vi "Simulated_Robot_Diff_Drive.vi"() -> ()   [LabVIEW 2019]
doc: "This WebSockets API example VI acts as a server for an incoming websockets connection. Receives/sends string data to the connected client."
uses:
  <vilib>/Rock Robotics/WPI/Simulation/Protocol/Devices/PWM/PWM proto.ctl
  <vilib>/Rock Robotics/WPI/Simulation/Protocol/Devices/PWM/PWM data proto.ctl
  <vilib>/Rock Robotics/WPI/Simulation/Protocol/Devices/RoboRIO/RoboRIO proto.ctl
  <vilib>/Rock Robotics/WPI/Simulation/Protocol/Devices/RoboRIO/RoboRIO data proto.ctl
  <vilib>/Rock Robotics/WPI/Simulation/Protocol/Devices/DriverStation/DS proto.ctl
  <vilib>/Rock Robotics/WPI/Simulation/Protocol/Devices/DriverStation/DS data proto.ctl
  <vilib>/Rock Robotics/WPI/Simulation/Protocol/Devices/Gyro/Gyro proto.ctl
  <vilib>/Rock Robotics/WPI/Simulation/Protocol/Devices/Gyro/Gyro Data proto.ctl
  <vilib>/Rock Robotics/WPI/Simulation/Protocol/Devices/Encoder/Encoder proto.ctl
  <vilib>/Rock Robotics/WPI/Simulation/Protocol/Devices/Encoder/Encoder data protoo.ctl
  <vilib>/Rock Robotics/WPI/ThirdParty/JAS_Junk/TrajLib/TypeDef/DIFF_DRIVE_TRAIN_SIM.ctl
  <vilib>/Rock Robotics/WPI/ThirdParty/JAS_Junk/TrajLib/TypeDef/LINEAR_SYSTEM.ctl
  <vilib>/Analysis/Matrix/Datatypes/RealMatrix.ctl
  <vilib>/Rock Robotics/WPI/ThirdParty/JAS_Junk/TrajLib/TypeDef/DCMOTOR.CTL
  <vilib>/vision/Image Controls.llb/IMAQ Image.ctl
  Simulated_Field/Simulated_Field_ROBOT_PICTURE.ctl
  DiffDriveSim/DiffDriveSim_PhysRobotInfoType.ctl
  DiffDriveSim/DiffDriveSim_KitBotDriveInfoType.ctl
  <vilib>/Rock Robotics/WPI/ThirdParty/JAS_Junk/TrajLib/Enum/DIFF_DRIVE_ToughBoxMini_MotorChoice_ENUM.ctl
  <vilib>/Rock Robotics/WPI/ThirdParty/JAS_Junk/TrajLib/Enum/DIFF_DRIVE_KitBot_WheelSize_ENUM.ctl
  <vilib>/Rock Robotics/WPI/ThirdParty/JAS_Junk/TrajLib/Enum/DIFF_DRIVE_ToughBoxMini_GearChoice_ENUM.ctl
  DiffDriveSim/DiffDriveSim_CustomDriveIntoType.ctl
  <vilib>/Rock Robotics/WPI/ThirdParty/JAS_Junk/TrajLib/Enum/DCMOTOR_TYPES_ENUM.ctl
  DiffDriveSim/DiffDriveSim_EncoderDIOType.ctl
  <vilib>/Rock Robotics/SystemInterfaces/DIO/FPGA_DIOChannel.ctl
  <vilib>/Rock Robotics/SystemInterfaces/DIO/FPGA_DIOPWMChannel.ctl
  <vilib>/Utility/miscctls.llb/LVBoundsTypeDef.ctl
  <vilib>/Rock Robotics/WPI/Simulation/Protocol/Devices/RoboRIO/RoboRIO Update Ops.ctl
  <vilib>/Rock Robotics/WPI/Simulation/Protocol/Devices/DriverStation/DS Update Ops.ctl
  <vilib>/Rock Robotics/WPI/ThirdParty/JAS_Junk/TrajLib/Rotation2d_CreateAngle.vi
  <vilib>/Rock Robotics/WPI/ThirdParty/JAS_Junk/TrajLib/Translation2d_Create.vi
  <vilib>/Rock Robotics/WPI/ThirdParty/JAS_Junk/TrajLib/MathUtil_Clamp.vi
  <vilib>/MediaMongrels Ltd/WebSockets/WebSockets/WebSocket Server/WebSocket Server.lvclass
  C:/Program Files/National Instruments/LabVIEW 2019/vi.lib/MediaMongrels Ltd/WebSockets/WebSockets/WebSocket/WebSocket.lvclass
  <vilib>/picture/pixmap.llb/Flatten Pixmap.vi
  <vilib>/picture/pictutil.llb/Create Mask.vi
  <vilib>/picture/picture.llb/Draw Flattened Pixmap.vi
  Simulated_Field/Simulated_Field.lvlib
  <vilib>/Rock Robotics/WPI/ThirdParty/JAS_Junk/TrajLib/Trajectory_Library.lvlib
  <vilib>/Analysis/Matrix/NI_Matrix.lvlib
panel:
  in  "Tab Control":T1(tab)
  in  "Start Simulation":bool
  in  "Field Selector":string(combo)
  in  "Robot Y Position\nInches":dbl=84.0
  in  "Robot X Position\nInches":dbl=120.0
  in  "Robot Orientation\nDegrees":dbl
  in  "Custom Drive Info":T2={"Motor Type"=enum."CIM", "Num Motors Per Side"=1, "Wheel Diameter Inch"=7.0, "Gear Ratio"=1.0} {"Gear Ratio" format="%#_13g"; "Wheel Diameter Inch" format="%#_13g"}
  in  "Robot Physical Info":T4={"Mass_LB"=80.0, "Actual TrackWidth Inch"=26.0, "Skid Factor"=1.75} {"Actual TrackWidth Inch" format="%#_13g"}
  in  "KitBot Drive Info":T5={"ToughBoxMiniMotor"=enum."One CIM Per Side", "Wheelsize"=enum."6 Inch", "ToughBoxMiniGear"=enum."Ratio_8_45"}
  in  "Use Custom Drive":bool
  in  "Encoder Counts/Rev":dbl=360.0
  in  "Left Drive Encoder":T9={"Enc A DI Channel"=enum."DIO 4", "Enc B DI Channel"=enum."DIO 5"}
  in  "Right Drive Encoder":T9={"Enc A DI Channel"=enum."DIO 6", "Enc B DI Channel"=enum."DIO 7"}
  in  "Left Drive Motor":T11
  in  "Right Drive Motor":T11=enum."PWM 1"
  out "Right Dist Ft":dbl format="%15.1f"
  out "Left Dist Ft":dbl format="%15.1f"
  out "Heading Deg":dbl format="%11.1f"
  out "Right Wheel\nFt / Sec":dbl format="%11.1f"
  out "Left Wheel\nFt / Sec":dbl format="%11.1f"
  out "RSL ON":picture
  out "ROBOT":T12
  out "RSL OFF":picture
  out "Field Picture":picture
  out "Y Pos Inch":dbl format="%11.1f"
  out "X Pos Inch":dbl format="%11.1f"
  out "Gyro":T13={"type"="Gyro", "device"="", "name"="", "data"={"<init"=0, ">connected"=FALSE, "<offsetX"=0.0, "<offsetY"=0.0, "<offsetZ"=0.0, ">angle_x"=0.0, ">angle_y"=0.0, ">angle_z"=0.0, ">rate_x"=0.0, ">rate_y"=0.0, ">rate_z"=0.0, "<gain"=0.0}}
  out "Enc Left":T15={"type"="Encoder", "device"="", "name"="", "data"={"<init"=FALSE, ">count"=0.0, ">period"=0.0, "<samples_to_avg"=0, "<offset"=0.0, "<channel_a"=0, "<channel_b"=0}}
  out "Enc Right":T15={"type"="Encoder", "device"="", "name"="", "data"={"<init"=FALSE, ">count"=0.0, ">period"=0.0, "<samples_to_avg"=0, "<offset"=0.0, "<channel_a"=0, "<channel_b"=0}}
  out "PWM 0":T17
  out "PWM 1":T17
  out "roboRIO":T19={"type"="roboRIO", "device"="", "name"="", "data"={">fpga_button"=FALSE, ">vin_voltage"=0.0, ">vin_current"=0.0, ">6v_voltage"=0.0, ">6v_current"=0.0, ">6v_active"=FALSE, ">6v_faults"=0.0, ">5v_voltage"=0.0, ">5v_current"=0.0, ">5v_active"=FALSE, ">5v_faults"=0.0, ">3v3_voltage"=0.0, ">3v3_current"=0.0, ">3v3_active"=FALSE, ">3v3_faults"=0.0}}
  out "Driverstation":T21={"type"="Driverstation", "device"="", "name"="", "data"={">enabled"=FALSE, ">autonomous"=FALSE, ">test"=FALSE, ">estop"=FALSE, ">fms"=FALSE, ">ds"=FALSE, "<match_time"=0.0, ">station"="", ">game_data"=""}}
  out "Request URI":string
  out "HTTP Headers":variant
  out "Stop Sim":bool
  out "Battery Voltage VDC":dbl format="%18.2f"
  out "Gyro Reading   Deg":dbl format="%19.3f"
  out "Edges/Feet":dbl
  out "out DiffDriveTrainSim":T23 {"m_Motor"."Jr_KgM2" format="%13.5p"; "m_Motor"."L_H" format="%13.5p"; "m_Motor"."Kt_NMPerAmp" format="%13.5p"; "m_Motor"."KvINV_RadPerSecPerVolt" format="%13.5p"; "m_Motor"."R_Ohms" format="%13.5p"; "m_Motor"."FreeSpeed_RadPerSec" format="%13.5p"; "m_Motor"."FreeCurrent_Amps" format="%13.5p"; "m_Motor"."StallCurrent_Amps" format="%13.5p"; "m_Motor"."StallTorque_NM" format="%13.5p"; "m_Motor"."nominalVoltage_Volts" format="%13.5p"}
  out "Speed Left  Ft/Sec":dbl format="%13.2f"
  out "Speed Right  Ft/Sec":dbl format="%13.2f"
  out "Amps":dbl
  out "PWM 0 Rate":dbl format="%19.3f"
  out "PWM 1 Rate":dbl format="%19.3f"
  out "FIeld Image":T27
  out "Y Pos Pixel":dbl format="%11.1f"
  out "X Pos Pixel":dbl format="%11.1f"
  in  "Restart":bool
  out "Ctrl Loop Offset MS":dbl
  out "Robot Enabled":bool
  # "Robot Position"
  # "Robot Speed / Distance"
  # "<States, 1>"
  # "<Outputs, 1>"
  # "<Inputs, 1>"
  # "<Outputs, 1>"
  # "<States,States>"
  # "<States,Inputs>"
  # "<Outputs,States>"
  # "<Outputs,Inputs>"
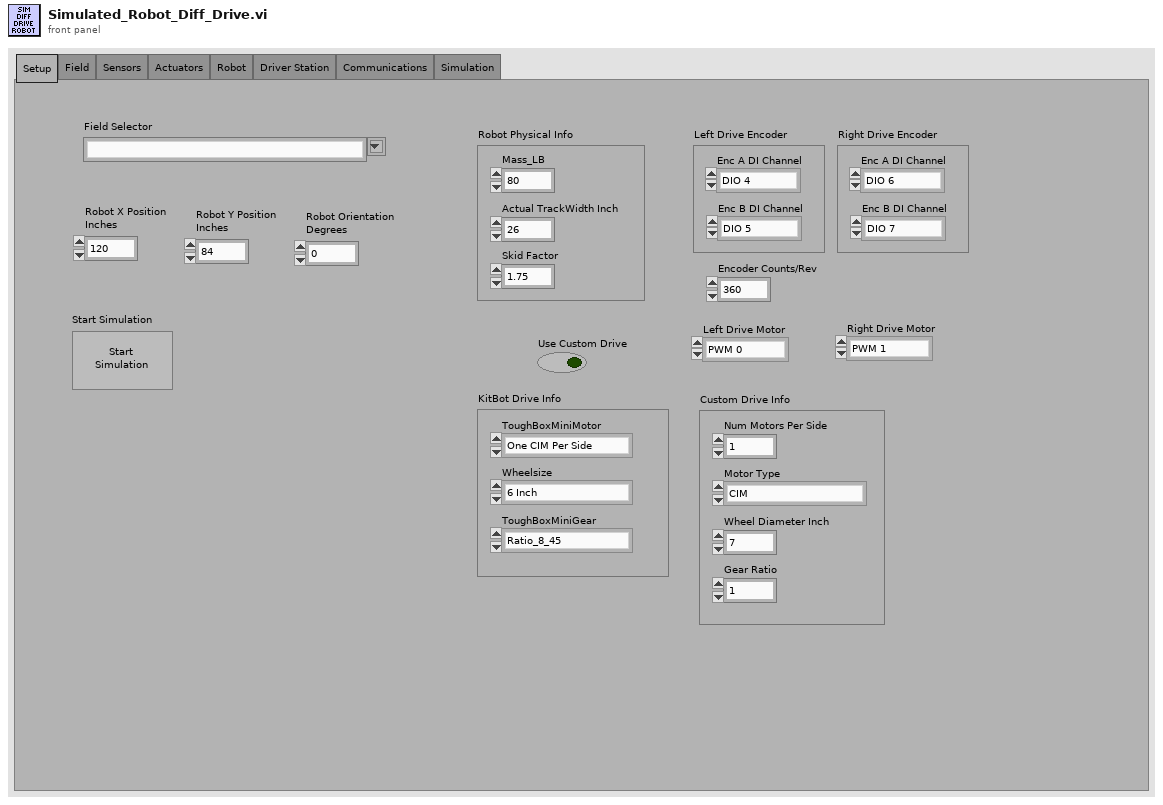
[diagram p1: front panel]
types:
  T1 = enum32{"Setup", "Field", "Sensors", "Actuators", "Robot", "Driver Station", "Communications", "Simulation"}
  T2 = typedef "DiffDriveSim_CustomDriveIntoType.ctl" = cluster{"Motor Type":T3, "Num Motors Per Side":i32, "Wheel Diameter Inch":dbl, "Gear Ratio":dbl}
  T3 = typedef "Trajectory_Library.lvlib/DCMOTOR_TYPES_ENUM.ctl" = enum16{"CIM", "AndyMark 9015", "Andy Mark RS 775 125", "Bag", "BaneBots RS 550", "BaneBots RS 775", "Falcon 500", "Mini CIM", "NEO", "NEO 550", "Romi BuiltIn", "Vex 775 Pro"}
  T4 = typedef "DiffDriveSim_PhysRobotInfoType.ctl" = cluster{"Mass_LB":dbl, "Actual TrackWidth Inch":dbl, "Skid Factor":dbl}
  T5 = typedef "DiffDriveSim_KitBotDriveInfoType.ctl" = cluster{"ToughBoxMiniMotor":T6, "Wheelsize":T7, "ToughBoxMiniGear":T8}
  T6 = typedef "Trajectory_Library.lvlib/DIFF_DRIVE_ToughBoxMini_MotorChoice_ENUM.ctl" = enum16{"One CIM Per Side", "Two CIM Per Side", "One MiniCIM Per Side", "Two Mini CIM Per Side", "Two Falcon Per Side", "Two NEO Per Side"}
  T7 = typedef "Trajectory_Library.lvlib/DIFF_DRIVE_KitBot_WheelSize_ENUM.ctl" = enum16{"4 Inch", "6 Inch", "8 Inch", "10 Inch"}
  T8 = typedef "Trajectory_Library.lvlib/DIFF_DRIVE_ToughBoxMini_GearChoice_ENUM.ctl" = enum16{"Ratio_12_75", "Ratio_10_71", "Ratio_8_45", "Ratio_7_31", "Ratio_5_95"}
  T9 = typedef "DiffDriveSim_EncoderDIOType.ctl" = cluster{"Enc A DI Channel":T10, "Enc B DI Channel":T10}
  T10 = typedef "FPGA_DIOChannel.ctl" = enum8{"DIO 0", "DIO 1", "DIO 2", "DIO 3", "DIO 4", "DIO 5", "DIO 6", "DIO 7", "DIO 8", "DIO 9", "DIO MXP 0", "DIO MXP 1", "DIO MXP 2", "DIO MXP 3", "DIO MXP 4", "DIO MXP 5", "DIO MXP 6", "DIO MXP 7", "DIO MXP 8", "DIO MXP 9", "DIO MXP 10", "DIO MXP 11", "DIO MXP 12", "DIO MXP 13", "DIO MXP 14", "DIO MXP 15", "SPI Port CS1", "SPI Port CS2", "SPI Port CS3", "SPI Port MISO", "SPI Port MOSI", "Invalid"}
  T11 = typedef "FPGA_DIOPWMChannel.ctl" = enum8{"PWM 0", "PWM 1", "PWM 2", "PWM 3", "PWM 4", "PWM 5", "PWM 6", "PWM 7", "PWM 8", "PWM 9", "PWM MXP 0", "PWM MXP 1", "PWM MXP 2", "PWM MXP 3", "PWM MXP 4", "PWM MXP 5", "PWM MXP 6", "PWM MXP 7", "PWM MXP 8", "PWM MXP 9", "Invalid"}
  T12 = typedef "Simulated_Field.lvlib/Simulated_Field_ROBOT_PICTURE.ctl" = picture
  T13 = typedef "Gyro proto.ctl" = cluster{"type":string, "device":string, "name":string, "data":T14}
  T14 = typedef "Gyro Data proto.ctl" = cluster{"<init":i32, ">connected":bool, "<offsetX":dbl, "<offsetY":dbl, "<offsetZ":dbl, ">angle_x":dbl, ">angle_y":dbl, ">angle_z":dbl, ">rate_x":dbl, ">rate_y":dbl, ">rate_z":dbl, "<gain":dbl}
  T15 = typedef "Encoder proto.ctl" = cluster{"type":string, "device":string, "name":string, "data":T16}
  T16 = typedef "Encoder data protoo.ctl" = cluster{"<init":bool, ">count":dbl, ">period":dbl, "<samples_to_avg":i32, "<offset":dbl, "<channel_a":i32, "<channel_b":i32}
  T17 = typedef "PWM proto.ctl" = cluster{"type":string, "device":string, "name":string, "data":T18}
  T18 = typedef "PWM data proto.ctl" = cluster{"<init":bool, "<speed":dbl, "<position":dbl, "<raw":dbl, "<period_scale":dbl, "<zero_latch":bool, "<servo range":dbl}
  T19 = typedef "RoboRIO proto.ctl" = cluster{"type":string, "device":string, "name":string, "data":T20}
  T20 = typedef "RoboRIO data proto.ctl" = cluster{">fpga_button":bool, ">vin_voltage":dbl, ">vin_current":dbl, ">6v_voltage":dbl, ">6v_current":dbl, ">6v_active":bool, ">6v_faults":dbl, ">5v_voltage":dbl, ">5v_current":dbl, ">5v_active":bool, ">5v_faults":dbl, ">3v3_voltage":dbl, ">3v3_current":dbl, ">3v3_active":bool, ">3v3_faults":dbl}
  T21 = typedef "DS proto.ctl" = cluster{"type":string, "device":string, "name":string, "data":T22}
  T22 = typedef "DS data proto.ctl" = cluster{">enabled":bool, ">autonomous":bool, ">test":bool, ">estop":bool, ">fms":bool, ">ds":bool, "<match_time":dbl, ">station":string, ">game_data":string}
  T23 = typedef "Trajectory_Library.lvlib/DIFF_DRIVE_TRAIN_SIM.ctl" = cluster{"m_Plant":T24, "m_X":T25, "m_Y":T25, "m_U":T25, "MeasureStdDev":T25, "m_Motor":T26, "m_OriginalGearing":dbl, "m_CurrentGearing":dbl, "m_WheelRadius_M":dbl, "m_RB":dbl}
  T24 = typedef "Trajectory_Library.lvlib/LINEAR_SYSTEM.ctl" = cluster{"m_A":T25, "m_B":T25, "m_C":T25, "m_D":T25, "States":i32, "Inputs":i32, "Outputs":i32}
  T25 = typedef "NI_Matrix.lvlib/RealMatrix.ctl" = dbl[][]
  T26 = typedef "Trajectory_Library.lvlib/DCMOTOR.CTL" = cluster{"nominalVoltage_Volts":dbl, "StallTorque_NM":dbl, "StallCurrent_Amps":dbl, "FreeCurrent_Amps":dbl, "FreeSpeed_RadPerSec":dbl, "R_Ohms":dbl, "KvINV_RadPerSecPerVolt":dbl, "Kt_NMPerAmp":dbl, "L_H":dbl, "Jr_KgM2":dbl}
  T27 = typedef "IMAQ Image.ctl" = refnum<image>
  T28 = typedef "LVBoundsTypeDef.ctl" = cluster{"Width":u32, "Height":u32}
  T29 = typedef "Image Type" = u32
  T30 = typedef "Simulated_Field.lvlib/Simulated_Field_Field_Info.ctl" = cluster{"FIeld_File_Name":string, "Top_Left_X":i32, "Top_Left_Y":i32, "Bottom_Right_X":i32, "Bottom_Right_Y":i32, "Field_Size_X":dbl, "Field_Size_Y":dbl, "FIeld_Size_Units":string}
  T31 = typedef "Trajectory_Library.lvlib/POSE2D.ctl" = cluster{"TRANSLATION":T32, "ROTATION":T33}
  T32 = typedef "Trajectory_Library.lvlib/TRANSLATION2D.ctl" = cluster{"X":dbl, "Y":dbl}
  T33 = typedef "Trajectory_Library.lvlib/ROTATION2D.ctl" = cluster{"VALUE":dbl, "COS":dbl, "SIN":dbl}
  T34 = typedef "Simulated_Field.lvlib/Simulated_FIeld_Rotated_Picture_TypeDef.ctl" = cluster{"ONE-8-bit pixmap":u8[][], "Two-Array":cdb[][], "Three-Numeric":i32, "Four-Numeric":i32, "Five-Numeric":cdb, "Six-colors":u32[], "Seven-new element/subarray":u32, "Eight-Cluster":cluster{"[0]":i32, "[1]":i32}}
  T35 = typedef "DS Update Ops.ctl" = enum16{"set enabled", "set autonomous", "set test", "set estop", "set fms", "set ds", "set control word", "set match_time", "set station", "set game data", "JSON update", "set name", "get", "transmit initial", "reset"}
  T36 = typedef "RoboRIO Update Ops.ctl" = enum16{"get", "JSON update", "set name", "transmit initial", "set fpga_button", "set vin_voltage", "set vin_current", "set 6v_voltage", "set 6v_current", "set 6v_active", "set 6v_faults", "set 5v_voltage", "set 5v_current", "set 5v_active", "set 5v_faults", "set 3v3_voltage", "set 3v3_current", "set 3v3_active", "set 3v3_faults", "reset"}
  T37 = cluster{"Right Speed Ft/Sec":dbl, "Right Distance Ft":dbl}
  T38 = cluster{"Left Speed Ft/Sec":dbl, "Left Distance Ft":dbl}
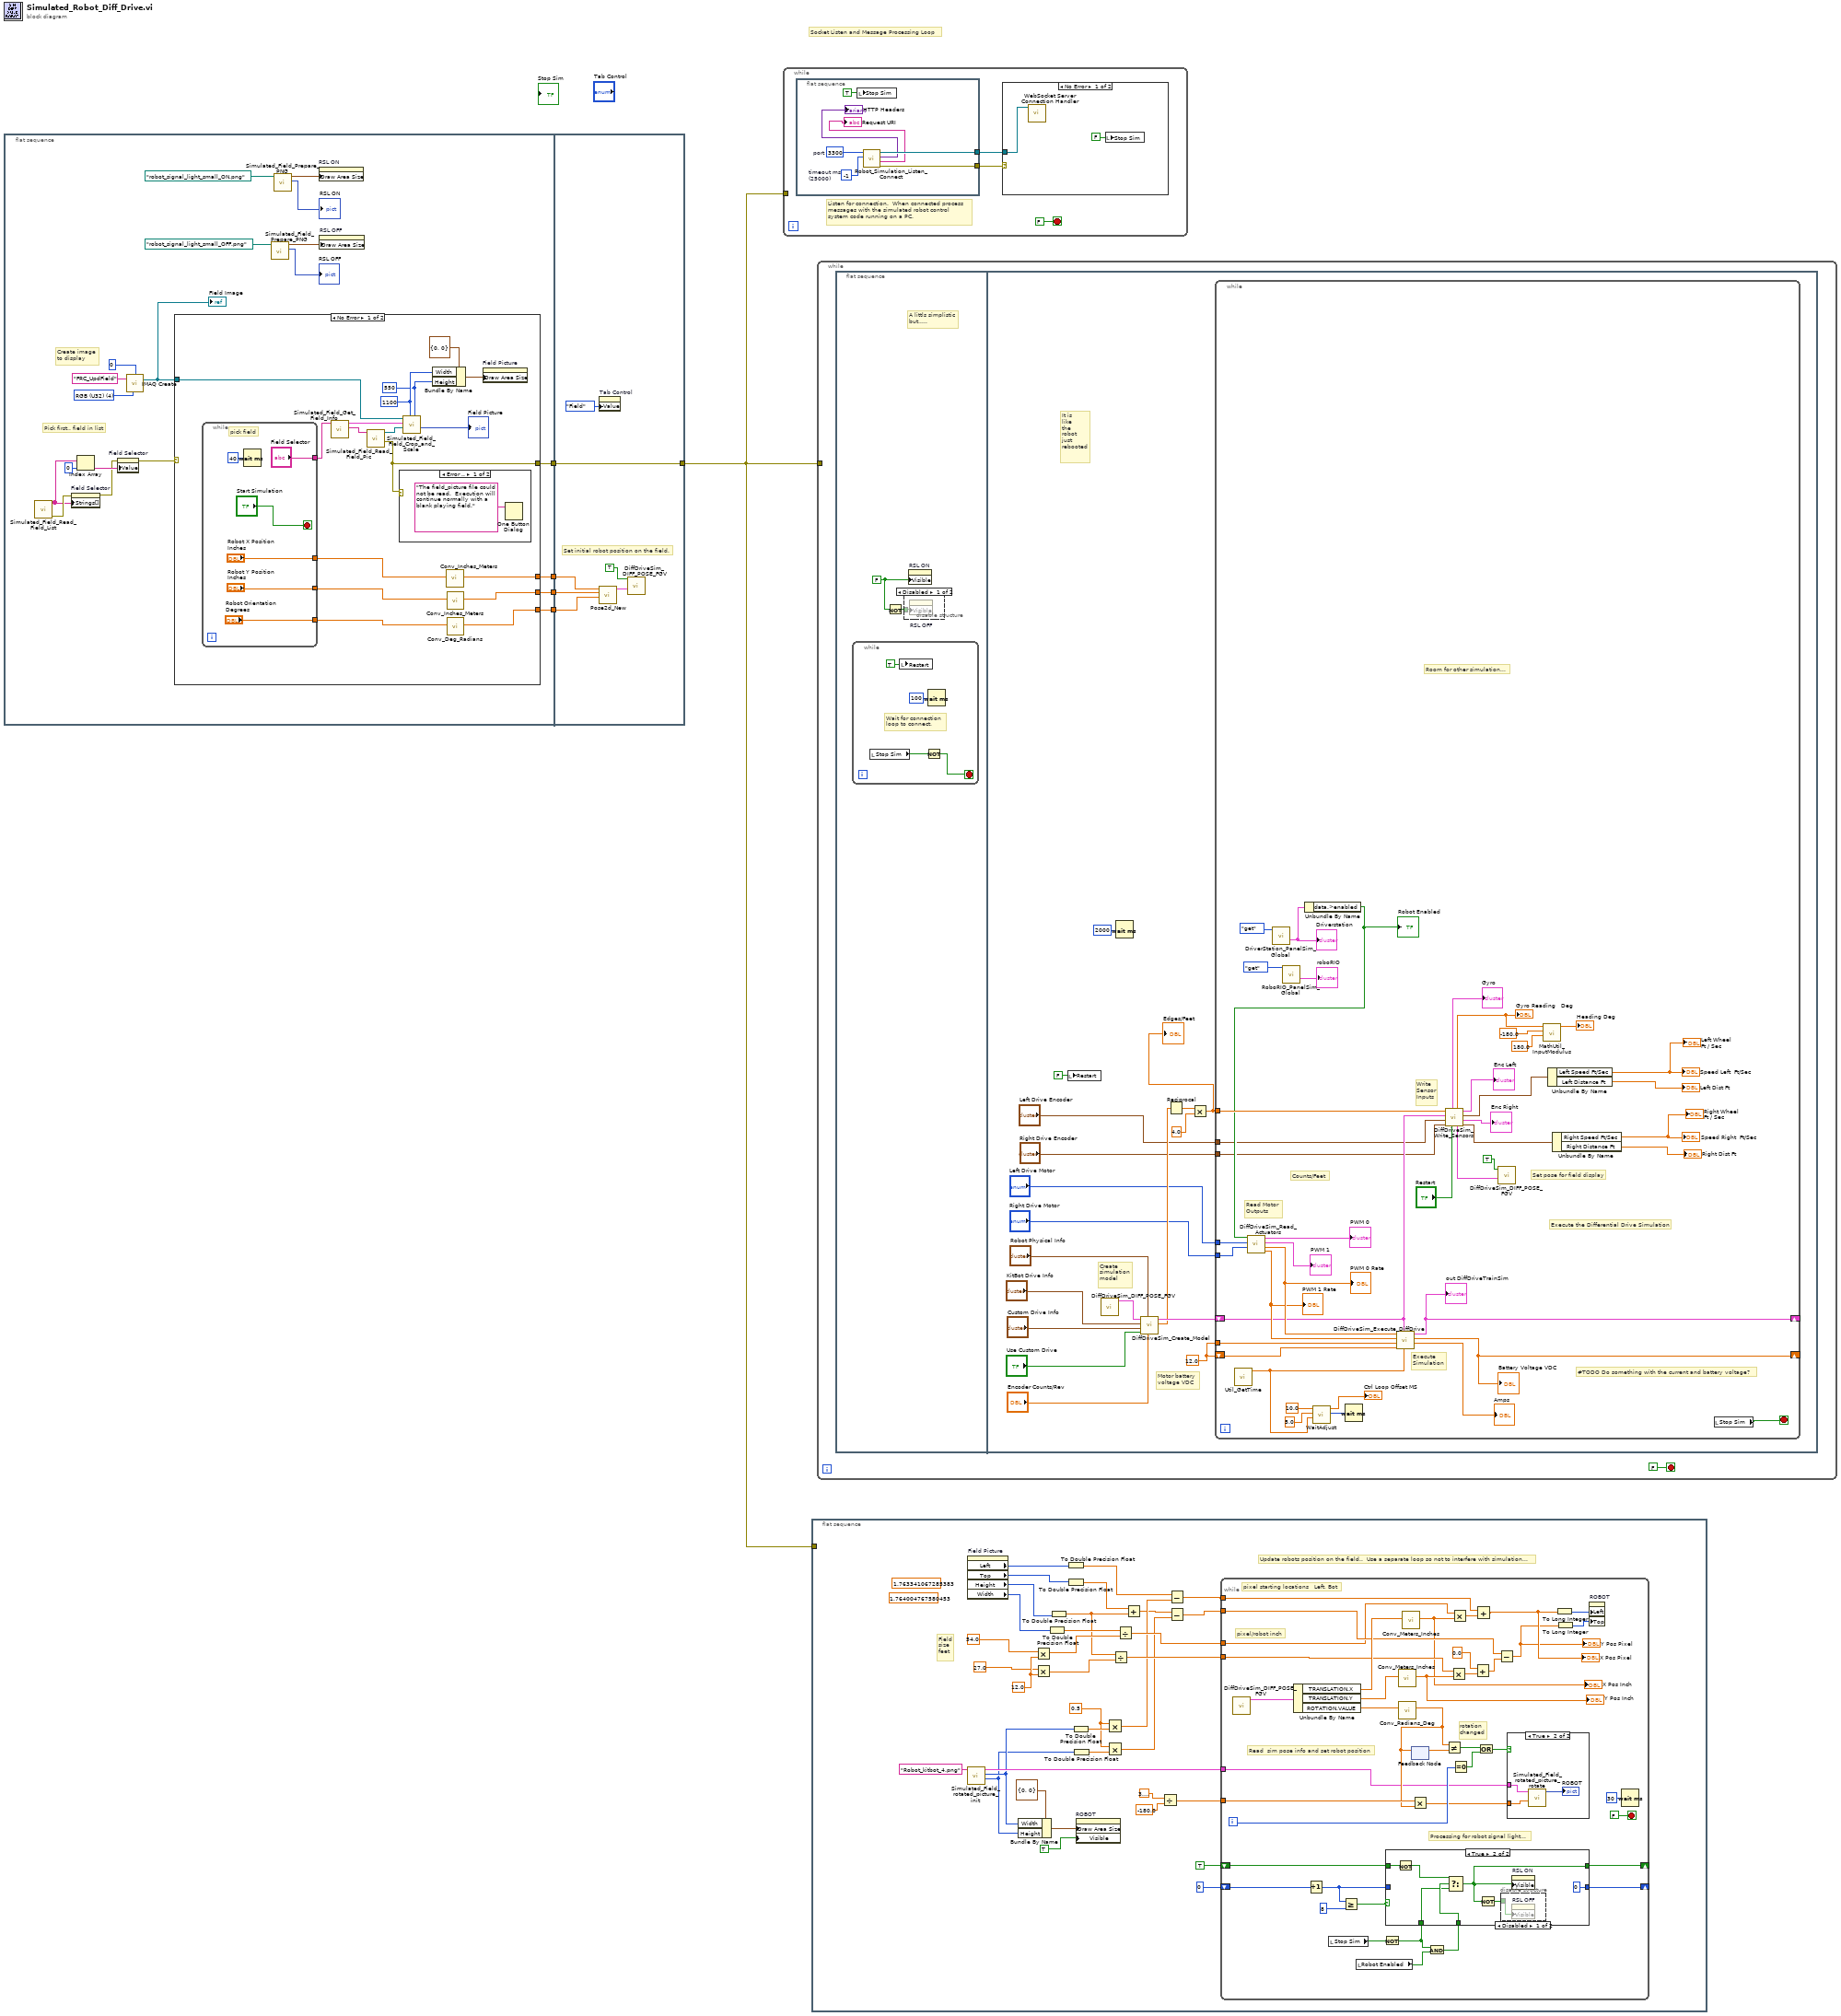
[diagram p0: block diagram]
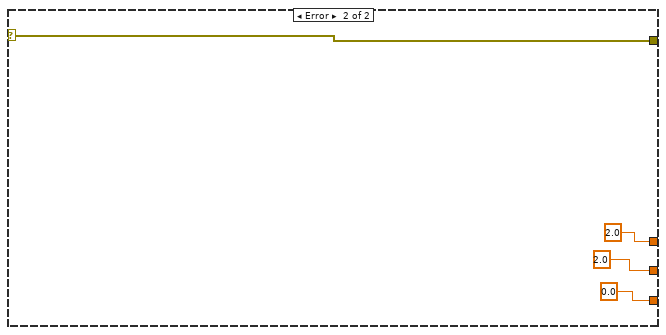
[diagram p6: hidden frame]
diagram:
  # "Socket Listen and Message Processing Loop"
  n1 = flat-sequence {
    tunnel: [w18] -> w5
    tunnel: [w8] -> w3
    tunnel: [w7] -> w2
    tunnel: [w6] -> w1
    tunnel: [w60] -> w4
    tunnel: w5 -> [w60]
    tunnel: w3 -> [w56]
    tunnel: w2 -> [w55]
    tunnel: w1 -> [w54]
    frame #0 {
      w23 = T29 4 items=["Grayscale (U8)", "Grayscale (I16)", "Grayscale (SGL)", "Complex (CSG)", "RGB (U32)", "HSL (U32)", "RGB (U64)", "Grayscale (U16)"] ("Image Type")
      # "Pick first.. field in list"
      # "Create image \nto display"
      n2 = call "Simulated_Field_Read_Field_List.vi"() -> ("error out"=w14:errorcluster, "section names"=w13:string[])  [unwired: 10 in]
      n3 = property on="Field Selector" class="CmbBox"(error in=w14, "Strings[]"=w13) -> (error out=w10:errorcluster)  [unwired: 1 in, 1 out]
      n4 = Index Array(array=w13, index=0) -> (element=w11:string)
      n5 = property on="Field Selector" class="CmbBox"(error in=w10, "Value"=w11) -> (error out=w9:errorcluster)  [unwired: 1 in, 1 out]
      n6 = call "IMAQ Create"("Border Size"=0, "Image Name"="FRC_UpdField", "Image Type"=w23) -> ("New Image"=w22:T27)  [unwired: 2 in, 1 out]
      "FIeld Image" <- w22
      n7 = case shown="No Error" w9 {
        selector: w9 -> [_ w53]
        tunnel: w22 -> [w33 _]
        tunnel: [w39 w53] -> w18
        tunnel: [w28 2.0 ("Meters")] -> w8
        tunnel: [w27 2.0 ("Meters")] -> w7
        tunnel: [w26 0.0 ("Radians")] -> w6
        frame No Error {
          w34 = 550 ("Disp Y Size Pixel")
          w35 = 1100 ("Disp X Size Pixel")
          n8 = while {
            tunnel: ["Field Selector"] -> w32
            tunnel: ["Robot X Position\nInches"] -> w31
            tunnel: ["Robot Y Position\nInches"] -> w30
            tunnel: ["Robot Orientation\nDegrees"] -> w29
            stop <- "Start Simulation" stop-if-true
            # "pick field"
            n9 = Wait (ms)(milliseconds to wait=u32 40) -> ()  [unwired: 1 out]
          }
          n10 = call "Simulated_Field_Get_Field_Info.vi"("Field Selector"=w32) -> ("File"=w42:string, "input cluster"=w41:T30)  [unwired: 9 in]
          n11 = call "Simulated_Field_Read_Field_Pic.vi"("file name"=w42) -> ("Image Error"=w39:errorcluster, "Image Data"=w40:T27)  [unwired: 7 in, 2 out]
          n12 = case shown="Error .." w39 {
            frame Error {
              n13 = One Button Dialog(message="The field_picture file could not be read.  Execution will continue normally with a blank playing field.") -> ()  [unwired: 1 in, 1 out]
            }
            frame No Error {
            }
          }
          n14 = call "Simulated_Field_Field_Crop_and_Scale.vi"("Disp Y Size Pixel"=w34, "Disp X Size Pixel"=w35, "Field Image"=w40, "field Info"=w41, "Display Image"=w33) -> ("Cropped Field Picture Out"=→"Field Picture":picture)  [unwired: 4 in, 2 out]
          n15 = Bundle By Name(cluster=T28 {"Width"=0, "Height"=0} ("Draw Area Size"), "Width"=w35, "Height"=w34) -> (w36:T28)
          n16 = call <vilib>:"Conv_Inches_Meters.vi"("INCH"=w31) -> ("Meters"=w28:dbl)  [unwired: 10 in]
          n17 = call <vilib>:"Conv_Inches_Meters.vi"("INCH"=w30) -> ("Meters"=w27:dbl)  [unwired: 10 in]
          n18 = call <vilib>:"Conv_Deg_Radians.vi"("Degress"=w29) -> ("Radians"=w26:dbl)  [unwired: 10 in]
          n19 = property on="Field Picture" class="Pict"("Draw Area Size"=w36) -> ()  [unwired: 2 in, 2 out]
        }
        frame Error {
        }
      }
      n20 = call "Simulated_Field_Prepare_PNG.vi"("path to PNG file"=path "robot_signal_light_small_OFF.png") -> ("new picture"=→"RSL OFF":picture, "Draw Area Size"=w17:T28)  [unwired: 9 in]
      n21 = call "Simulated_Field_Prepare_PNG.vi"("path to PNG file"=path "robot_signal_light_small_ON.png") -> ("new picture"=→"RSL ON":picture, "Draw Area Size"=w20:T28)  [unwired: 9 in]
      n22 = property on="RSL ON" class="Pict"("Draw Area Size"=w20) -> ()  [unwired: 2 in, 2 out]
      n23 = property on="RSL OFF" class="Pict"("Draw Area Size"=w17) -> ()  [unwired: 2 in, 2 out]
    }
    frame #1 {
      # "Set initial robot position on the field."
      n24 = property on="Tab Control" class="TabCtl (strict)"("Value"=T1."Field" ("Tab Control")) -> ()  [unwired: 2 in, 2 out]
      n25 = call <vilib>:"Pose2d_New.vi"("Heading"=w54, "Y"=w55, "X"=w56) -> ("out POSe"=w59:T31)  [unwired: 8 in]
      n26 = call "DiffDriveSim_DIFF_POSE_FGV.vi"("in Sim Pose"=w59, "WRITE"=TRUE) -> ()  [unwired: 9 in, 1 out]
    }
  }
  n27 = while {
    tunnel: w4 -> [_]
    stop <- FALSE stop-if-true
    # "Listen for connection.  When connected process\nmessages with the simulated robot control\nsystem code running on a PC."
    n28 = flat-sequence {
      tunnel: [w68] -> w62
      tunnel: [w66] -> w61
      frame #0 {
        w69 = -1  # timeout ms  (25000)
        w70 = u16 3300  # port
        n29 = local write "Stop Sim"(TRUE ("Stop\nSim")) -> ()
        n30 = call <vilib>:"Robot_Simulation_Listen_Connect.vi"("timeout ms (25000)"=w69, "port"=w70) -> ("error out"=w68:errorcluster, "Properties:Request URI"=→"Request URI":string, "Properties:Return Headers"=→"HTTP Headers":variant, "WebSocket Connection out"=w66:refnum<class "WebSocket Server.lvclass">)  [unwired: 6 in]
      }
    }
    n31 = case shown="No Error" w62 {
      tunnel: w61 -> [w71 _]
      frame No Error {
        n32 = call <vilib>:"WebSocket Server Connection Handler.vi"("WebSocket in"=w71) -> ()  [unwired: 10 in, 1 out]
        n33 = local write "Stop Sim"(FALSE ("Stop\nSim")) -> ()
      }
      frame Error {
      }
    }
  }
  n34 = flat-sequence {
    tunnel: w4 -> [_]
    frame #0 {
      w85 = 0.5
      (unwired) 1.764004767580453
      (unwired) 1.763341067285383
      w103 = 12.0 ("y")
      # "Field\nsize\nfeet"
      # "Update robots position on the field..  Use a separate loop so not to interfere with simulation..."
      n35 = call "Simulated_Field_rotated_picture_init.vi"("Picture FIle Name"="Robot_kitbot_4.png") -> ("Height"=w77:i16, "Width"=w78:i16, "RotatedPictureInfo"=w104:T34)  [unwired: 7 in, 1 out]
      n36 = property on="Field Picture" class="Pict"() -> ("Left"=w100:i32, "Top"=w99:i32, "Height"=w98:u32, "Width"=w97:u32)  [unwired: 2 in, 2 out]
      n37 = Bundle By Name(cluster=T28 {"Width"=0, "Height"=0} ("Draw Area Size"), "Width"=w78, "Height"=w77) -> (w80:T28)
      n38 = Multiply(x=54.0, y=w103) -> (x*y=w94:dbl)
      n39 = Multiply(x=27.0, y=w103) -> (x*y=w91:dbl)
      n40 = To Double Precision Float(number=w97) -> (double precision float=w95:dbl)
      n41 = To Double Precision Float(number=w98) -> (double precision float=w92:dbl)
      n42 = To Double Precision Float(number=w100) -> (double precision float=w84:dbl)
      n43 = To Double Precision Float(number=w99) -> (double precision float=w96:dbl)
      n44 = To Double Precision Float(number=w78) -> (double precision float=w87:dbl)
      n45 = To Double Precision Float(number=w77) -> (double precision float=w86:dbl)
      n46 = property on="ROBOT" class="Pict (strict)"("Draw Area Size"=w80, "Visible"=TRUE) -> ()  [unwired: 2 in, 2 out]
      n47 = Multiply(x=w85, y=w87) -> (x*y=w83:dbl)
      n48 = Multiply(x=w85, y=w86) -> (x*y=w81:dbl)
      n49 = Divide(x=w92, y=w91) -> (x/y=w90:dbl)
      n50 = Divide(x=w95, y=w94) -> (x/y=w93:dbl)
      n51 = Add(x=w96, y=w92) -> (x+y=w82:dbl)
      n52 = Divide(x=3.141592653589793, y=-180.0 ("value")) -> (x/y=w107:dbl)
      n53 = Subtract(x=w84, y=w83) -> (x-y=w89:dbl)
      n54 = Subtract(x=w82, y=w81) -> (x-y=w88:dbl)
      n55 = while {
        tunnel: w107 -> [w147]
        tunnel: w104 -> [w130]
        tunnel: w89 -> [w129]
        tunnel: w88 -> [w128]
        tunnel: w93 -> [w127]
        tunnel: w90 -> [w126]
        shift-right: [w112] -> _
        shift-left: 0 -> [w115]
        shift-right: [w113] -> _
        shift-left: TRUE -> [w114]
        i -> [w136]
        stop <- FALSE stop-if-true
        # "Processing for robot signal light..."
        # "pixel starting locations   Left, Bot"
        # "Read  sim pose info and set robot position"
        # "pixel/robot inch"
        # "rotation\nchanged"
        n56 = call "DiffDriveSim_DIFF_POSE_FGV.vi"() -> ("out Sim Pose"=w119:T31)  [unwired: 11 in]
        n57 = Unbundle By Name(w119) -> ("TRANSLATION.X"=w135:dbl, "TRANSLATION.Y"=w134:dbl, "ROTATION.VALUE"=w132:dbl)
        n58 = Increment(x=w115) -> (x+1=w117:i32)
        n59 = local read "Stop Sim"() -> (w109:bool)
        n60 = Greater Or Equal?(x=w117, y=8) -> (x >= y?=w118:bool)
        n61 = local read "Robot Enabled"() -> (w110:bool)
        n62 = Not(x=w109) -> (.not. x?=w108:bool)
        n63 = call <vilib>:"Conv_Meters_Inches.vi"("Meters"=w134) -> ("Inches"=w121:dbl)  [unwired: 10 in]
        "Y Pos Inch" <- w121
        n64 = call <vilib>:"Conv_Radians_Deg.vi"("Radians"=w132) -> ("Degrees"=w133:dbl)  [unwired: 10 in]
        n65 = call <vilib>:"Conv_Meters_Inches.vi"("Meters"=w135) -> ("Inches"=w120:dbl)  [unwired: 10 in]
        "X Pos Inch" <- w120
        n66 = feedback-in #1(w133) -> ()
        n67 = feedback #1() -> (w144:dbl)  [unwired: 1 in]
        n68 = Multiply(x=w147, y=w133) -> (x*y=w131:dbl)
        n69 = And(x=w108, y=w110) -> (x .and. y?=w111:bool)
        n70 = case shown="True" w118 {
          tunnel: w114 -> [w149 w156]
          tunnel: [w149 w152] -> w113
          tunnel: w117 -> [w148 _]
          tunnel: [w148 0] -> w112
          tunnel: w111 -> [_ w154]
          tunnel: w108 -> [_ w150]
          frame False {
          }
          frame True {
            n71 = Not(x=w156) -> (.not. x?=w155:bool)
            n72 = Select(t=w155, s=w154, f=w150) -> (s? t:f=w152:bool)
            n73 = Not(x=w152) -> (.not. x?=w153:bool)
            n74 = disable-structure shown="Disabled" {
              disable-tunnel: w153 -> [w157 _]
              frame Disabled {
                n75 = property on="RSL OFF" class="Pict"("Visible"=w157) -> ()  [unwired: 2 in, 2 out]
              }
              frame Enabled {
              }
            }
            n76 = property on="RSL ON" class="Pict"("Visible"=w152) -> ()  [unwired: 2 in, 2 out]
          }
        }
        n77 = Not Equal?(x=w133, y=w144) -> (x != y?=w138:bool)
        n78 = Multiply(x=w126, y=w121) -> (x*y=w142:dbl)
        n79 = Multiply(x=w127, y=w120) -> (x*y=w143:dbl)
        n80 = Equal To 0?(x=w136) -> (x = 0?=w137:bool)
        n81 = Add(x=0.0, y=w142) -> (x+y=w140:dbl)
        n82 = Add(x=w129, y=w143) -> (x+y=w123:dbl)
        "X Pos Pixel" <- w123
        n83 = Or(x=w138, y=w137) -> (x .or. y?=w139:bool)
        n84 = Subtract(x=w128, y=w140) -> (x-y=w122:dbl)
        "Y Pos Pixel" <- w122
        n85 = case shown="True" w139 {
          tunnel: w131 -> [_ w158]
          tunnel: w130 -> [_ w159]
          frame False {
          }
          frame True {
            n86 = call "Simulated_Field_rotated_picture_rotate.vi"("Angle"=w158, "RotatedPictureInfo"=w159) -> ("new picture"=→"ROBOT":picture)  [unwired: 9 in]
          }
        }
        n87 = To Long Integer(number=w123) -> (32bit integer=w125:i32)
        n88 = To Long Integer(number=w122) -> (32bit integer=w124:i32)
        n89 = property on="ROBOT" class="Pict (strict)"("Left"=w125, "Top"=w124) -> ()  [unwired: 2 in, 2 out]
        n90 = Wait (ms)(milliseconds to wait=u32 30) -> ()  [unwired: 1 out]
      }
    }
  }
  n91 = while {
    tunnel: w4 -> [_]
    stop <- FALSE stop-if-true
    n92 = flat-sequence {
      frame #0 {
        w162 = FALSE ("Visible")
        # "A littls simplistic\nbut....."
        n93 = while {
          stop <- w166 stop-if-true
          # "Wait for connection\nloop to connect."
          n94 = local read "Stop Sim"() -> (w167:bool)
          n95 = local write "Restart"(TRUE ("Restart")) -> ()
          n96 = Not(x=w167) -> (.not. x?=w166:bool)
          n97 = Wait (ms)(milliseconds to wait=u32 100) -> ()  [unwired: 1 out]
        }
        n98 = Not(x=w162) -> (.not. x?=w163:bool)
        n99 = disable-structure shown="Disabled" {
          disable-tunnel: w163 -> [w164 _]
          frame Disabled {
            n100 = property on="RSL OFF" class="Pict"("Visible"=w164) -> ()  [unwired: 2 in, 2 out]
          }
          frame Enabled {
          }
        }
        n101 = property on="RSL ON" class="Pict"("Visible"=w162) -> ()  [unwired: 2 in, 2 out]
      }
      frame #1 {
        w185 = 12.0 ("Voltage")
        # "Create\nsimulation\nmodel"
        # "Motor battery\nvoltage VDC"
        # "It is\nlike\nthe \nrobot \njust\nrebooted"
        n102 = local write "Restart"(FALSE ("Restart")) -> ()
        n103 = call "DiffDriveSim_DIFF_POSE_FGV.vi"() -> ("out Sim Pose"=w184:T31)  [unwired: 11 in]
        n104 = Wait (ms)(milliseconds to wait=u32 2000) -> ()  [unwired: 1 out]
        n105 = call "DiffDriveSim_Create_Model.vi"("Encoder Counts/Rev"="Encoder Counts/Rev", "Robot Physical Info"="Robot Physical Info", "Use Custom Drive"="Use Custom Drive", "Custom Drive Info"="Custom Drive Info", "KitBot Drive Info"="KitBot Drive Info", "Initial Robot Position"=w184) -> ("Encoder Ft/Count"=w183:dbl, "out DiffDriveTrainSim"=w186:T23)  [unwired: 4 in]
        n106 = Reciprocal(x=w183) -> (1/x=w177:dbl)
        n107 = Multiply(x=w177, y=4.0) -> (x*y=w175:dbl)
        "Edges/Feet" <- w175
        n108 = while {
          shift-right: [w218] -> _
          shift-left: w186 -> [w212]
          shift-right: [w217] -> _
          shift-left: w185 -> [w210]
          tunnel: w175 -> [w216]
          tunnel: w185 -> [w211]
          tunnel: "Left Drive Encoder" -> [w202]
          tunnel: "Right Drive Encoder" -> [w201]
          tunnel: "Left Drive Motor" -> [w199]
          tunnel: "Right Drive Motor" -> [w198]
          stop <- w222 stop-if-true
          # "Room for other simulation..."
          # "Execute\nSimulation"
          # "Write\nSensor\nInputs"
          # "Read Motor\nOutputs"
          # "#TODO Do something with the current and battery voltage?"
          # "Counts/Feet"
          # "Set pose for field display"
          # "Execute the Differential Drive Simulation"
          n109 = call <vilib>:"Util_GetTime.vi"() -> ("FPGA_Time_Seconds"=w194:dbl)  [unwired: 10 in, 1 out]
          n110 = call <vilib>:"DriverStation_PanelSim_Global.vi"("menu"=DS_Update_Ops."get") -> ("Driverstation new"=w221:T21)  [unwired: 13 in, 1 out]
          "Driverstation" <- w221
          n111 = call <vilib>:"RoboRIO_PanelSim_Global.vi"("Menu"=RoboRIO_Update_Ops."get") -> ("roboRIO new"=→"roboRIO":T19)  [unwired: 13 in, 1 out]
          n112 = Unbundle By Name(w221) -> ("data.>enabled"=w214:bool)
          "Robot Enabled" <- w214
          n113 = call "DiffDriveSim_Read_Actuators.vi"("Right Drive Motor"=w198, "Left Drive Motor"=w199, "Robot Enabled"=w214) -> ("Right Motor Dmd"=w213:dbl, "Left Motor Dmd"=w215:dbl, "Right PWM Sim"=→"PWM 1":T17, "Left PWM Sim"=→"PWM 0":T17)  [unwired: 5 in]
          "PWM 0 Rate" <- w215
          "PWM 1 Rate" <- w213
          n114 = call <vilib>:"WaitAdjust.vi"("Time_SEC"=w194, "MaxDeviation_MS"=5.0, "DesiredLoopTime_MS"=10.0) -> ("AdjustedWaitTime_MS"=w195:u32, "Offset_MS"=→"Ctrl Loop Offset MS":dbl)  [unwired: 7 in]
          n115 = Wait (ms)(milliseconds to wait=w195) -> ()  [unwired: 1 out]
          n116 = call "DiffDriveSim_Execute_DiffDrive.vi"("Time"=w194, "in DiffDriveTrainSim"=w212, "Actual  Battery Voltage"=w210, "Nominal Battery Voltage"=w211, "Right Motor Dmd"=w213, "Left Motor Dmd"=w215) -> ("Current Amps"=→"Amps":dbl, "Battery Volts"=w217:dbl, "out DiffDriveTrainSim"=w218:T23)  [unwired: 3 in]
          "out DiffDriveTrainSim" <- w218
          "Battery Voltage VDC" <- w217
          n117 = call "DiffDriveSim_Write_Sensors.vi"("Restart"="Restart", "Right Encoder"=w201, "Left Encoder"=w202, "Diff Drive Train Sim"=w212, "Counts/Feet"=w216) -> (0:"Right Encoder"=w191:T37, 1:"Right Encoder"=→"Enc Right":T15, 2:"Left Encoder"=w192:T38, 3:"Left Encoder"=→"Enc Left":T15, "Robot Pose"=w209:T31, "Gyro Deg"=w206:dbl, "Gyro"=→"Gyro":T13)
          "Gyro Reading   Deg" <- w206
          n118 = call "DiffDriveSim_DIFF_POSE_FGV.vi"("in Sim Pose"=w209, "WRITE"=TRUE) -> ()  [unwired: 9 in, 1 out]
          n119 = call <vilib>:"MathUtil_InputModulus.vi"("Maximum_Input"=180.0, "Minimum_Input"=-180.0, "Input"=w206) -> ("modulus"=→"Heading Deg":dbl)  [unwired: 8 in]
          n120 = Unbundle By Name(w192) -> ("Left Speed Ft/Sec"=→"Speed Left  Ft/Sec" →"Left Wheel\nFt / Sec":dbl, "Left Distance Ft"=→"Left Dist Ft":dbl)
          n121 = Unbundle By Name(w191) -> ("Right Speed Ft/Sec"=→"Speed Right  Ft/Sec" →"Right Wheel\nFt / Sec":dbl, "Right Distance Ft"=→"Right Dist Ft":dbl)
          n122 = local read "Stop Sim"() -> (w222:bool)
        }
      }
    }
  }
